vi "BestYInverso.vi"(9 "atacando contra":bool, 10 "IA State":T1={"our_robots"=[], "enemy_robots"=[], "balls"=[], "geometry"={"line_width"=0, "field_length"=0, "field_width"=0, "boundary_width"=0, "referee_width"=0, "goal_width"=0, "goal_depth"=0, "goal_wall_width"=0, "center_circle_radius"=0, "defense_radius"=0, "defense_stretch"=0, "free_kick_from_defense_dist"=0, "penalty_spot_from_field_line_dist"=0, "penalty_line_from_spot_dist"=0}, "IA Judge"={"stage"="", "command"="", "our_goalie_id"=0.0, "enemy_goalie_id"=0.0, "command enum"=enum."Halt", "Time"=enum."Azul"}, "Received Timestamp"=timestamp(0 s since 1904-01-01), "Events"={"Touch"=FALSE, "Ball out"=FALSE, "id touch"=0.0, "Ball out of \nVision"=FALSE, "Ball inside \nGoalie area"=FALSE, "Robot not responding"=FALSE, "Robots responding status"=[1.0, 1.0, 1.0, 1.0, 1.0, 1.0], "Enemy Ball \nPossession"=FALSE, "Pass State"=FALSE, "id end of pass"=0.0, "Kick"=FALSE, "Id Possession"=0.0}, "Position"=[]}) -> (1 "Position":dbl[](array[numeric]), 2 "IA State 2":T1={"our_robots"=[], "enemy_robots"=[], "balls"=[], "geometry"={"line_width"=0, "field_length"=0, "field_width"=0, "boundary_width"=0, "referee_width"=0, "goal_width"=0, "goal_depth"=0, "goal_wall_width"=0, "center_circle_radius"=0, "defense_radius"=0, "defense_stretch"=0, "free_kick_from_defense_dist"=0, "penalty_spot_from_field_line_dist"=0, "penalty_line_from_spot_dist"=0}, "IA Judge"={"stage"="", "command"="", "our_goalie_id"=0.0, "enemy_goalie_id"=0.0, "command enum"=enum."Halt", "Time"=enum."Azul"}, "Received Timestamp"=timestamp(0 s since 1904-01-01), "Events"={"Touch"=FALSE, "Ball out"=FALSE, "id touch"=0.0, "Ball out of \nVision"=FALSE, "Ball inside \nGoalie area"=FALSE, "Robot not responding"=FALSE, "Robots responding status"=[1.0, 1.0, 1.0, 1.0, 1.0, 1.0], "Enemy Ball \nPossession"=FALSE, "Pass State"=FALSE, "id end of pass"=0.0, "Kick"=FALSE, "Id Possession"=0.0}, "Position"=[]})   [LabVIEW 2016]
uses:
  Core/AI Input.ctl
  Core/AI Robot.ctl
  Intel/Functions Enum.ctl
  Intel/AttackerStates.ctl
  Core/AI Ball.ctl
  Core/Field Size.ctl
  Core/AI Judge.ctl
  Intel/Command Enum.ctl
  Events/Events.ctl
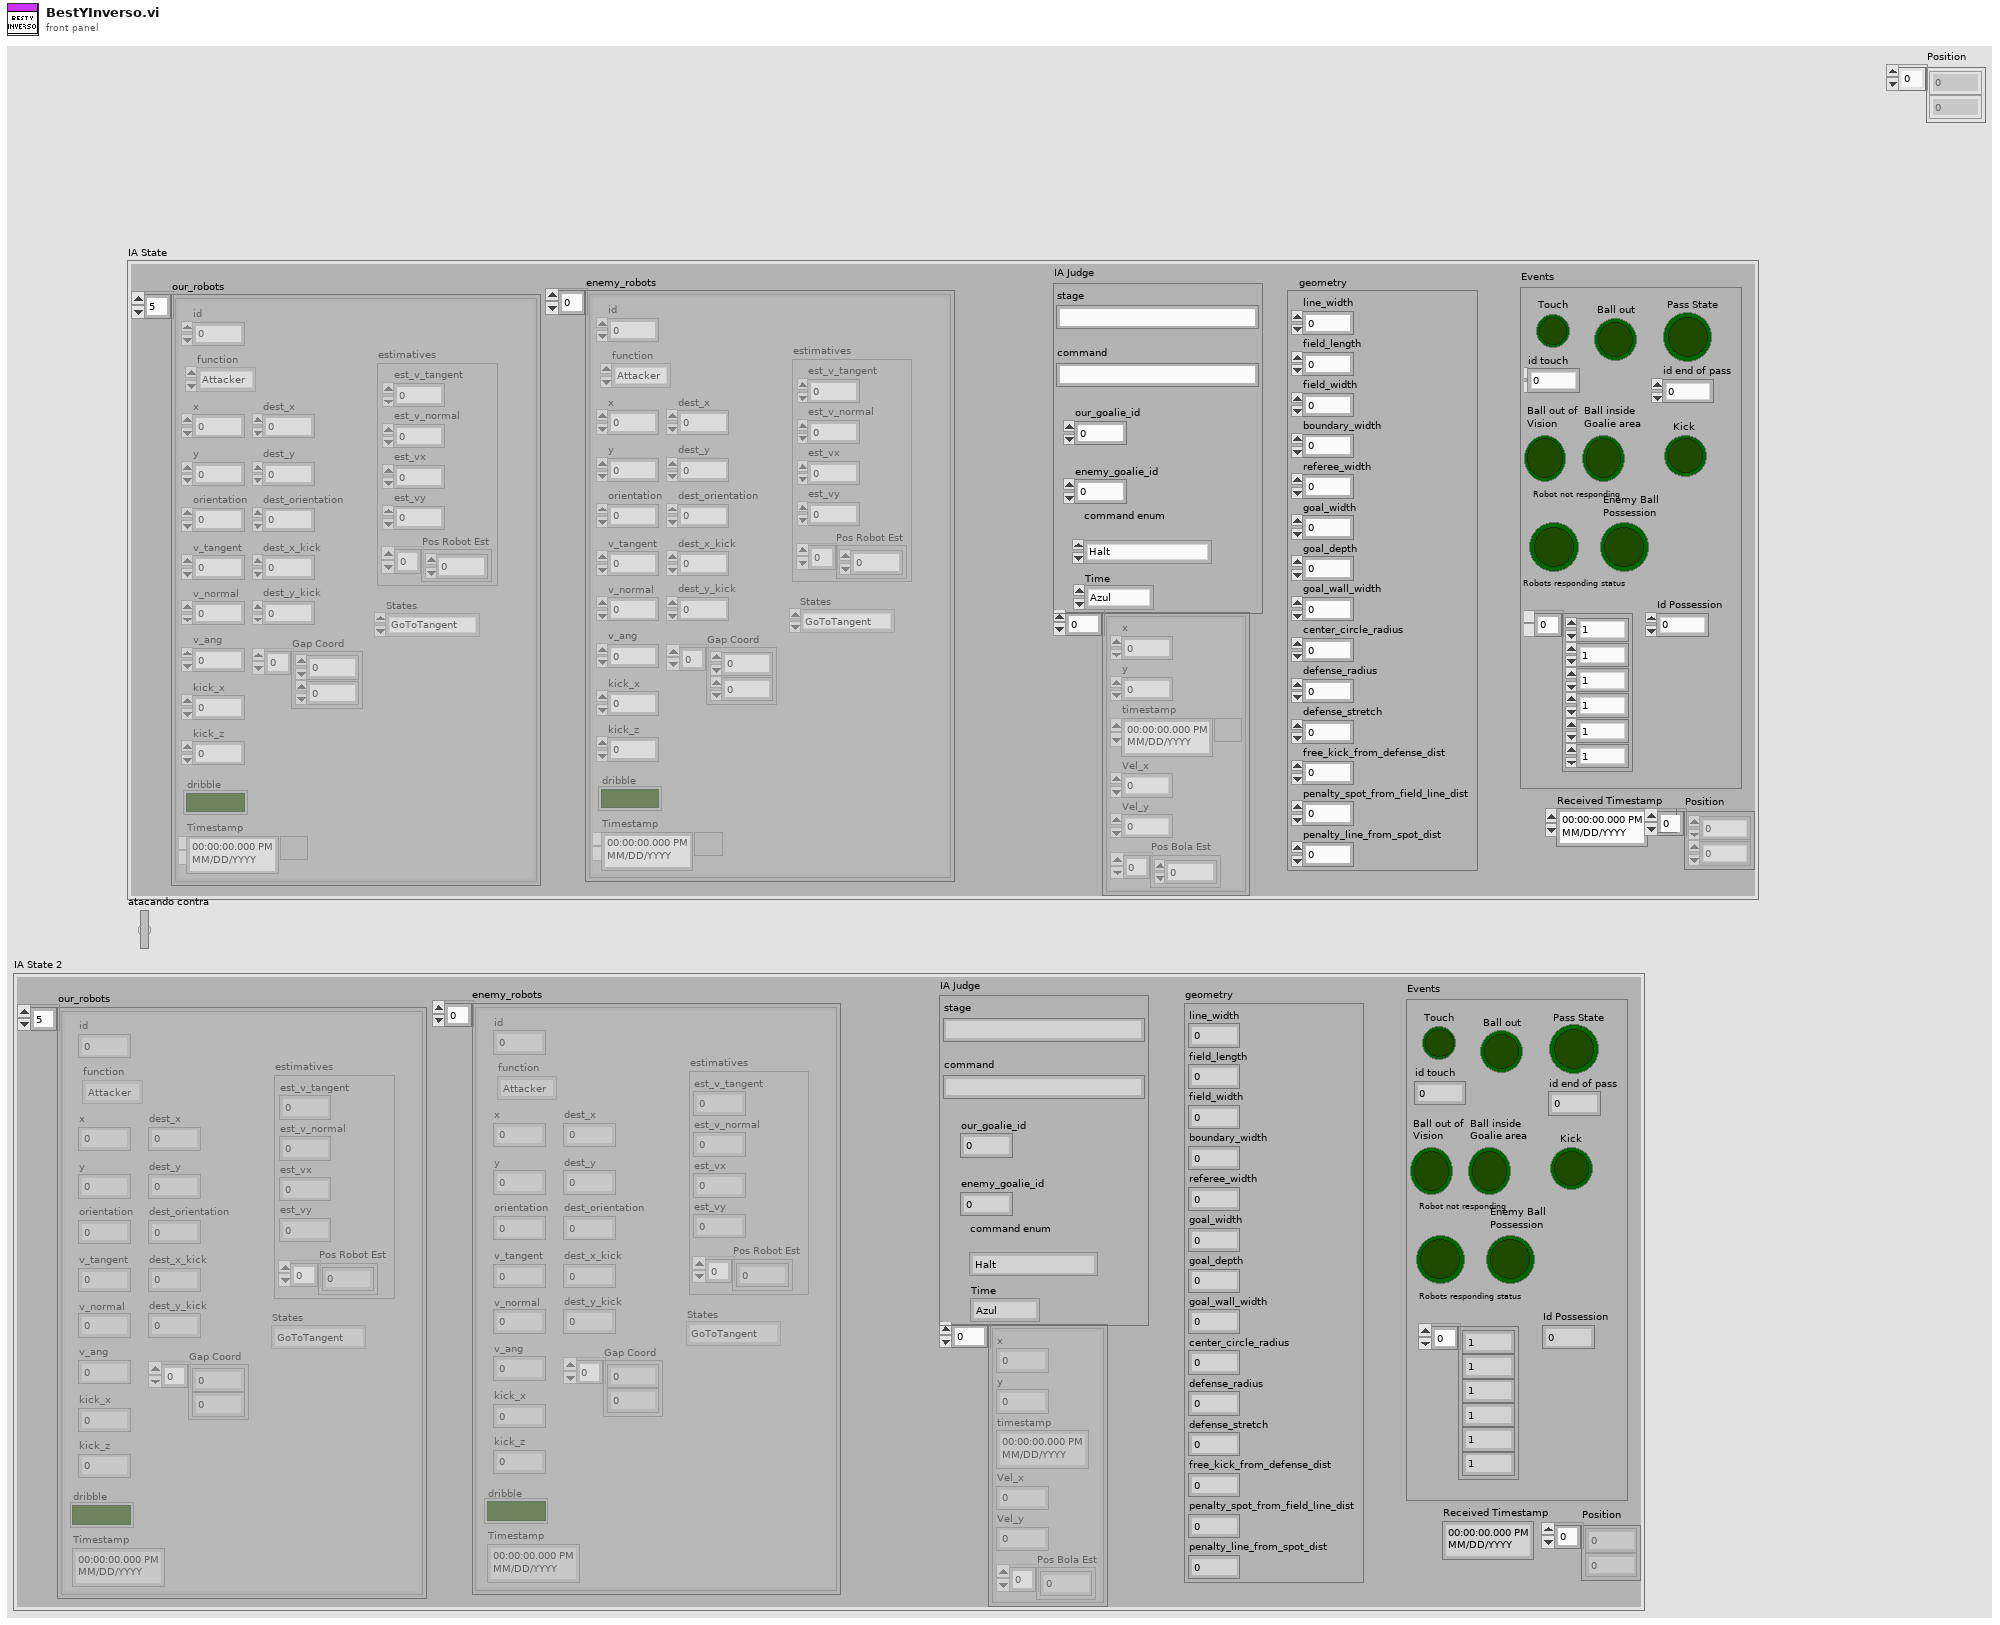
[diagram p1: front panel]
types:
  T1 = typedef "AI Input.ctl" = cluster{"our_robots":T2[], "enemy_robots":T2[], "balls":T5[], "geometry":T6, "IA Judge":T7, "Received Timestamp":timestamp, "Events":T9, "Position":dbl[]}
  T2 = typedef "AI Robot.ctl" = cluster{"id":u32, "function":T3, "x":dbl, "y":dbl, "orientation":dbl, "v_tangent":dbl, "v_normal":dbl, "v_ang":dbl, "kick_x":dbl, "kick_z":dbl, "dribble":bool, "Timestamp":timestamp, "dest_x":dbl, "dest_y":dbl, "dest_orientation":dbl, "estimatives":cluster{"est_v_tangent":dbl, "est_v_normal":dbl, "est_vx":dbl, "est_vy":dbl, "Pos Robot Est":dbl[]}, "dest_x_kick":dbl, "dest_y_kick":dbl, "Gap Coord":dbl[], "States":T4}
  T3 = typedef "Functions Enum.ctl" = enum16{"Attacker", "Goalie", "Defender", "Striker", "Goto 0", "Dummy", "Kicker", "ZigZag"}
  T4 = typedef "AttackerStates.ctl" = enum16{"Pass", "GoToTangent", "BallGetting", "GoToKick", ""}
  T5 = typedef "AI Ball.ctl" = cluster{"x":dbl, "y":dbl, "timestamp":timestamp, "Vel_x":dbl, "Vel_y":dbl, "Pos Bola Est":dbl[]}
  T6 = typedef "Field Size.ctl" = cluster{"line_width":u32, "field_length":u32, "field_width":u32, "boundary_width":u32, "referee_width":u32, "goal_width":u32, "goal_depth":u32, "goal_wall_width":u32, "center_circle_radius":u32, "defense_radius":u32, "defense_stretch":u32, "free_kick_from_defense_dist":u32, "penalty_spot_from_field_line_dist":u32, "penalty_line_from_spot_dist":u32}
  T7 = typedef "AI Judge.ctl" = cluster{"stage":string, "command":string, "our_goalie_id":dbl, "enemy_goalie_id":dbl, "command enum":T8, "Time":enum16{"Azul", "Amarelo"}}
  T8 = typedef "Command Enum.ctl" = enum16{"Halt", "Stop", "Force Start", "PKA Normal Start", "Prepare Kickoff Ally", "PKE Normal Start", "Prepare Kickoff Enemy", "Prepare Penalty Ally", "PPA Normal Start", "Prepare Penalty Enemy", "PPE Normal Start", "Direct Free Enemy", "Direct Free Ally", "Indirect Free Enemy", "Indirect Free Ally", "Timeout Enemy", "Timeout Ally", "Goal Enemy", "Goal Ally", "Ball Placement Enemy", "Ball Placement Ally", "Normal Half Time", "Extra Time Break", "Extra Half Time", "None"}
  T9 = typedef "Events.ctl" = cluster{"Touch":bool, "Ball out":bool, "id touch":dbl, "Ball out of \nVision":bool, "Ball inside \nGoalie area":bool, "Robot not responding":bool, "Robots responding status":dbl[], "Enemy Ball \nPossession":bool, "Pass State":bool, "id end of pass":dbl, "Kick":bool, "Id Possession":dbl}
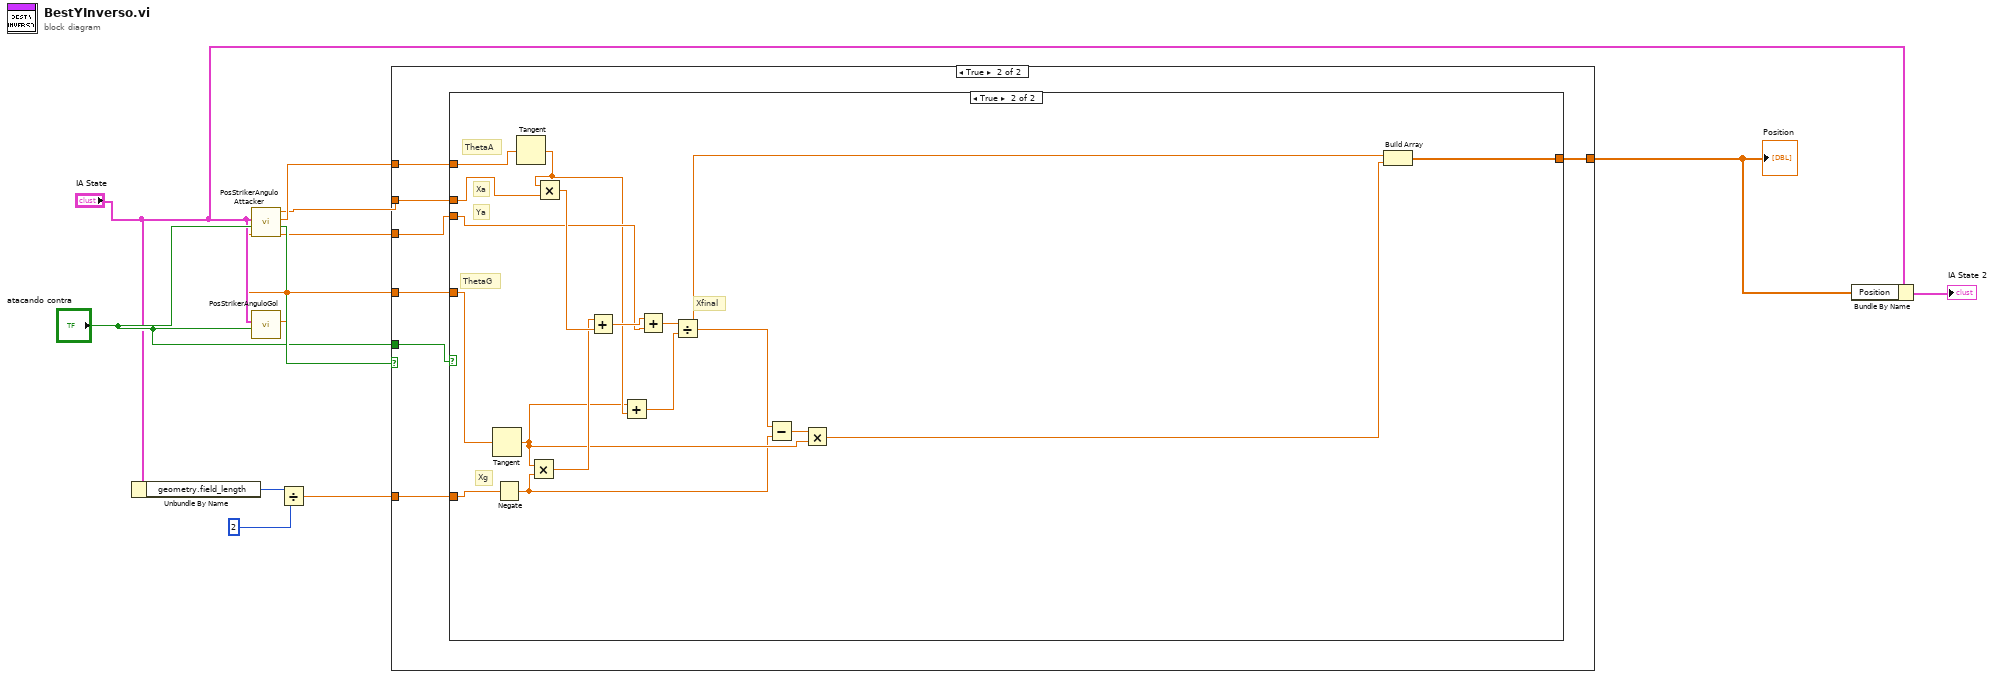
[diagram p0: block diagram]
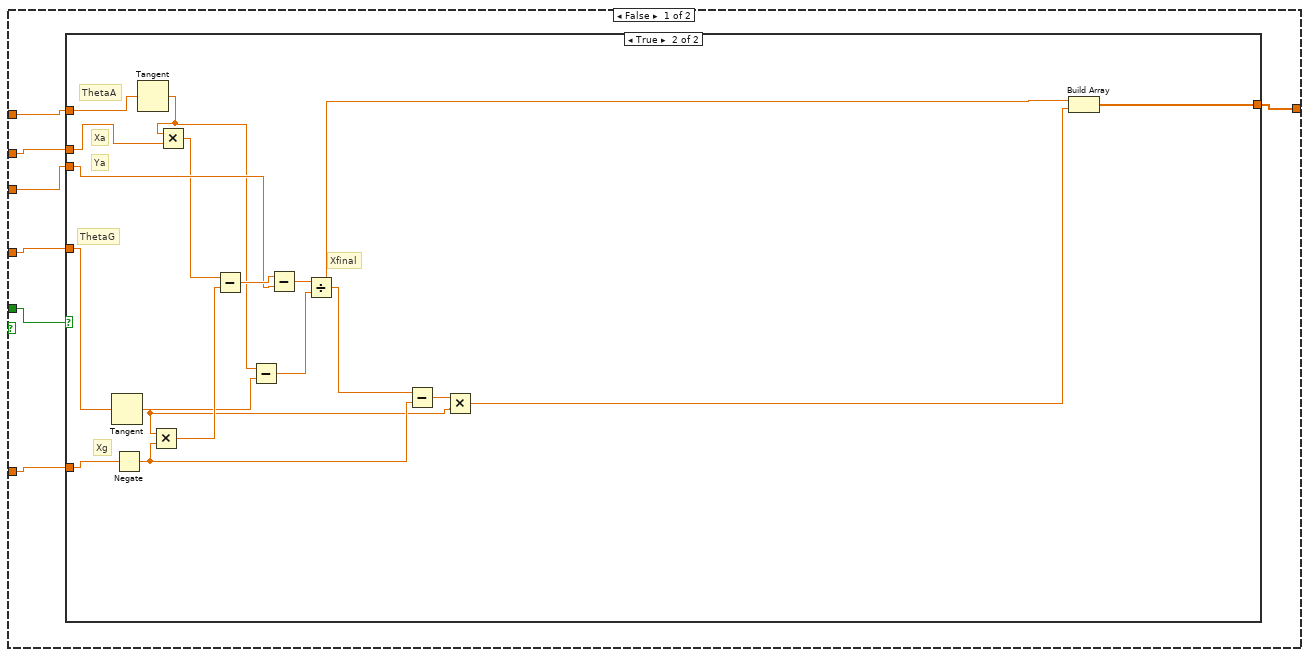
[diagram p2: hidden frame]
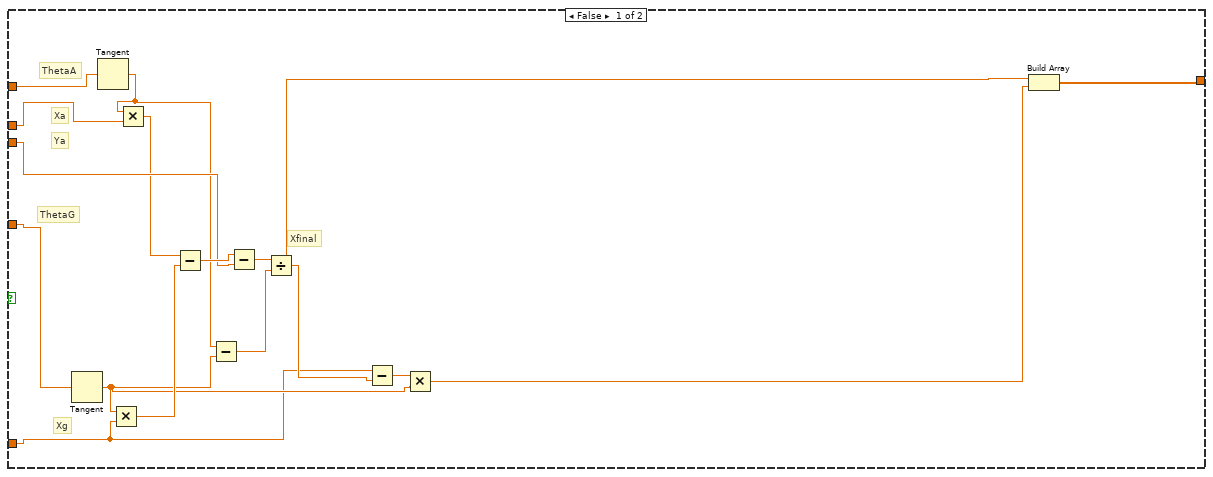
[diagram p3: hidden frame]
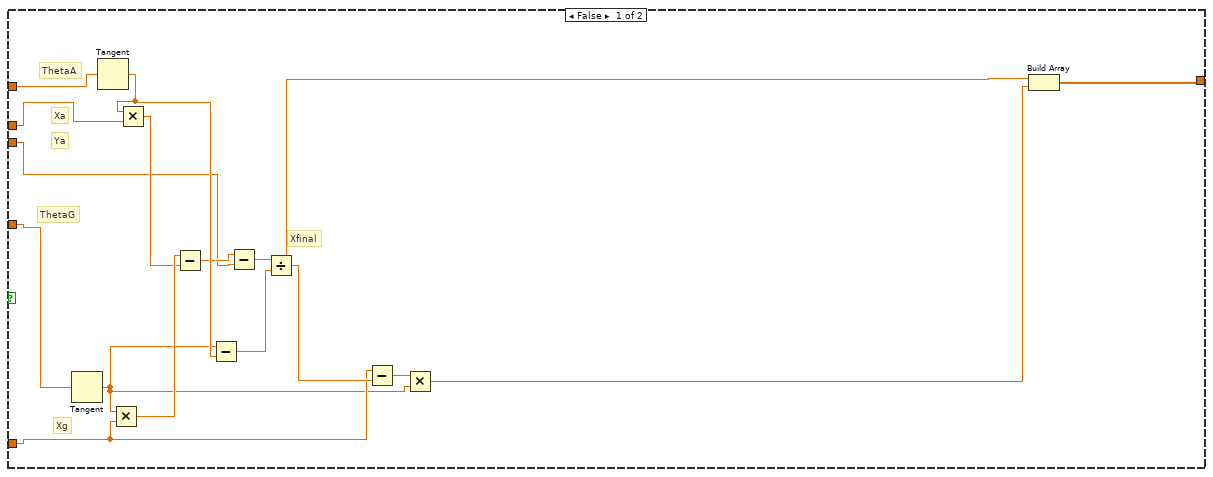
[diagram p4: hidden frame]
diagram:
  n1 = Unbundle By Name("IA State") -> ("geometry.field_length"=w7:u32)
  n2 = call "PosStrikerAnguloGol.vi"("atacando contra"="atacando contra", "IA State"="IA State") -> ("theta final"=w1:dbl)  [unwired: 9 in]
  n3 = call "PosStrikerAnguloAttacker.vi"("AnguloGol"=w1, "atacando contra"="atacando contra", "IA State"="IA State") -> ("YdoAttacker 2"=w8:dbl, "AttackerPositive?"=w12:bool, "theta final"=w10:dbl, "XdoAttacker 2"=w9:dbl)  [unwired: 5 in]
  n4 = Divide(x=w7, y=u32 2) -> (x/y=w5:dbl)
  n5 = case shown="True" w12 {
    tunnel: "atacando contra" -> [w13 w59]
    tunnel: w10 -> [w18 w58]
    tunnel: w9 -> [w17 w57]
    tunnel: w8 -> [w16 w56]
    tunnel: w1 -> [w15 w55]
    tunnel: w5 -> [w14 w54]
    tunnel: [w19 w53] -> w2
    frame False {
      n6 = case shown="True" w13 {
        tunnel: w18 -> [w29 w49]
        tunnel: w17 -> [w28 w50]
        tunnel: w16 -> [w27 w47]
        tunnel: w15 -> [w30 w51]
        tunnel: w14 -> [w20 w52]
        tunnel: [w26 w42] -> w19
        frame False {
          # "Xfinal"
          # "Xg"
          # "ThetaG"
          # "Ya"
          # "Xa"
          # "ThetaA"
          n7 = Tangent(1:w30) -> (0:w22:dbl)
          n8 = Tangent(1:w29) -> (0:w23:dbl)
          n9 = Multiply(x=w22, y=w20) -> (x*y=w25:dbl)
          n10 = Multiply(x=w23, y=w28) -> (x*y=w24:dbl)
          n11 = Subtract(x=w24, y=w25) -> (x-y=w31:dbl)
          n12 = Subtract(x=w23, y=w22) -> (x-y=w33:dbl)
          n13 = Subtract(x=w31, y=w27) -> (x-y=w32:dbl)
          n14 = Divide(x=w32, y=w33) -> (x/y=w21:dbl)
          n15 = Subtract(x=w20, y=w21) -> (x-y=w34:dbl)
          n16 = Multiply(x=w34, y=w22) -> (x*y=w35:dbl)
          n17 = Build Array(w21, w35) -> (w26:dbl[])
        }
        frame True {
          # "Xfinal"
          # "Xg"
          # "ThetaG"
          # "Ya"
          # "Xa"
          # "ThetaA"
          n18 = Tangent(1:w51) -> (0:w36:dbl)
          n19 = Negate(x=w52) -> (-x=w41:dbl)
          n20 = Tangent(1:w49) -> (0:w37:dbl)
          n21 = Multiply(x=w36, y=w41) -> (x*y=w39:dbl)
          n22 = Multiply(x=w37, y=w50) -> (x*y=w38:dbl)
          n23 = Subtract(x=w38, y=w39) -> (x-y=w48:dbl)
          n24 = Subtract(x=w37, y=w36) -> (x-y=w45:dbl)
          n25 = Subtract(x=w48, y=w47) -> (x-y=w46:dbl)
          n26 = Divide(x=w46, y=w45) -> (x/y=w40:dbl)
          n27 = Subtract(x=w40, y=w41) -> (x-y=w44:dbl)
          n28 = Multiply(x=w44, y=w36) -> (x*y=w43:dbl)
          n29 = Build Array(w40, w43) -> (w42:dbl[])
        }
      }
    }
    frame True {
      n30 = case shown="True" w59 {
        tunnel: w58 -> [w65 w89]
        tunnel: w57 -> [w64 w90]
        tunnel: w56 -> [w63 w85]
        tunnel: w55 -> [w66 w91]
        tunnel: w54 -> [w62 w92]
        tunnel: [w61 w80] -> w53
        frame False {
          # "Xfinal"
          # "Xg"
          # "ThetaG"
          # "Ya"
          # "Xa"
          # "ThetaA"
          n31 = Tangent(1:w66) -> (0:w60:dbl)
          n32 = Tangent(1:w65) -> (0:w74:dbl)
          n33 = Multiply(x=w60, y=w62) -> (x*y=w68:dbl)
          n34 = Multiply(x=w74, y=w64) -> (x*y=w67:dbl)
          n35 = Subtract(x=w68, y=w67) -> (x-y=w69:dbl)
          n36 = Subtract(x=w60, y=w74) -> (x-y=w71:dbl)
          n37 = Subtract(x=w69, y=w63) -> (x-y=w70:dbl)
          n38 = Divide(x=w70, y=w71) -> (x/y=w72:dbl)
          n39 = Subtract(x=w62, y=w72) -> (x-y=w73:dbl)
          n40 = Multiply(x=w73, y=w60) -> (x*y=w75:dbl)
          n41 = Build Array(w72, w75) -> (w61:dbl[])
        }
        frame True {
          # "Xfinal"
          # "Xg"
          # "ThetaG"
          # "Ya"
          # "Xa"
          # "ThetaA"
          n42 = Tangent(1:w91) -> (0:w78:dbl)
          n43 = Negate(x=w92) -> (-x=w77:dbl)
          n44 = Tangent(1:w89) -> (0:w79:dbl)
          n45 = Multiply(x=w78, y=w77) -> (x*y=w87:dbl)
          n46 = Multiply(x=w79, y=w90) -> (x*y=w88:dbl)
          n47 = Add(x=w87, y=w88) -> (x+y=w86:dbl)
          n48 = Add(x=w78, y=w79) -> (x+y=w83:dbl)
          n49 = Add(x=w86, y=w85) -> (x+y=w84:dbl)
          n50 = Divide(x=w84, y=w83) -> (x/y=w76:dbl)
          n51 = Subtract(x=w76, y=w77) -> (x-y=w82:dbl)
          n52 = Multiply(x=w82, y=w78) -> (x*y=w81:dbl)
          n53 = Build Array(w76, w81) -> (w80:dbl[])
        }
      }
    }
  }
  "Position" <- w2
  n54 = Bundle By Name(cluster="IA State", "Position"=w2) -> (→"IA State 2":T1)
